vi "timestamp to string.vi"(7 "Return UTC":bool, 10 "Format":string(combo), 11 "time stamp":timestamp) -> (3 "date/time string":string)   [LabVIEW 2013]
panel:
  # "%^<%Y_%m_%d_T%H_%M_%S>T\n2011_01_11_T13_01_11\n%^<%Y_%m_%d_%H_%M_%S>T\n2011_01_11_13_01_11\n%^<%Y_%m_%d_T%H_%M_%S>T.txt\n2011_01_11_T13_01_11.txt\n\n%^<%b %d %Y %I:%M:%S %p>T\nJan 01 2012 01:01:11 PM\n%^<%b %d %Y %H:%M:%S>T\nJan 01 2012 13:01:11 \n%^<%a %d %b %Y %H:%M:%S>T\nSun 01 Jan 2012 13:01:11\n%^<%a %d %b %Y %I:%M:%S %p>T\nSun 01 Jan 2012 01:01:11 PM\n%^<%I:%M:%S %p %a %#m/%#d/%Y>T\n01:01:11 PM Sun 1/1/2012\n\n%^<%I:%M:%S %p>T\n01:01:11 PM\n%^<%H:%M:%S>T\n13:01:11\n%^<%a, %b %d %Y>T\nSun, Jan 01 2012\n%^<%d %b %Y>T\n01 Jan 2012"
  # "%^<%#I:%#M:%S %p %#m/%#d/%Y>T\n1:1:11 PM 1/11/2011 (USsmall TD)\n%^<%I:%M:%S %p %m/%d/%Y>T\n01:01:11 PM 01/11/2011 (USfull TD)\n\n%^<%#m/%#d/%Y %#I:%#M:%S %p>T\n1/11/2011 1:1:11 PM (USsmall DT)\n%^<%m/%d/%Y %I:%M:%S %p>T\n01/11/2011 01:01:11 PM(USfull DT)\n\n%^<%#H:%#M:%S %#d/%#m/%Y>T\n13:1:11 11/1/2011 (eurosmall TD)\n%^<%H:%M:%S %d/%m/%Y>T\n13:01:11 11/01/2011 (eurofull TD)\n\n%^<%#d/%#m/%Y %#H:%#M:%S>T\n13:1:11 11/1/2011 (eurosmall TD)\n%^<%d/%m/%Y %H:%M:%S>T\n13:01:11 11/01/2011 (eurofull TD)\n\n%^<%Y-%m-%d %H:%M:%S>T\n2011-11-01 13:01:11 (mysql datetime)"
  # "Time format codes have leading zeros as necessary to ensure a constant field width. An optional # modifier before the format code letter removes the leading zeros from the following format codes:\n\n%#d, %#H, %#I, %#j, %#m, %#M, %#s, %#S, %#U, %#w, %#W, %#X, %#y, %#Y\n\nDisplays a timestamp value or a numeric value as time in the format you specify using time format codes. For example, %c displays locale-specific date/time. Time-related format codes include the following: %X (locale-specific time), %H (hour, 24-hour clock), %I (hour, 12-hour clock), %M (minute), %S (second), %<digit>u (fractional seconds with <digit> precision), and %p (a.m./p.m. flag). Date-related format codes include the following: %x (locale-specific date), %y (year within century), %Y (year including century), %m (month number), %b (abbreviated month name), %d (day of month), and %a (abbreviated weekday name).\n%j day of year\n%W week of year\n%U full week of year\n%w day of week"
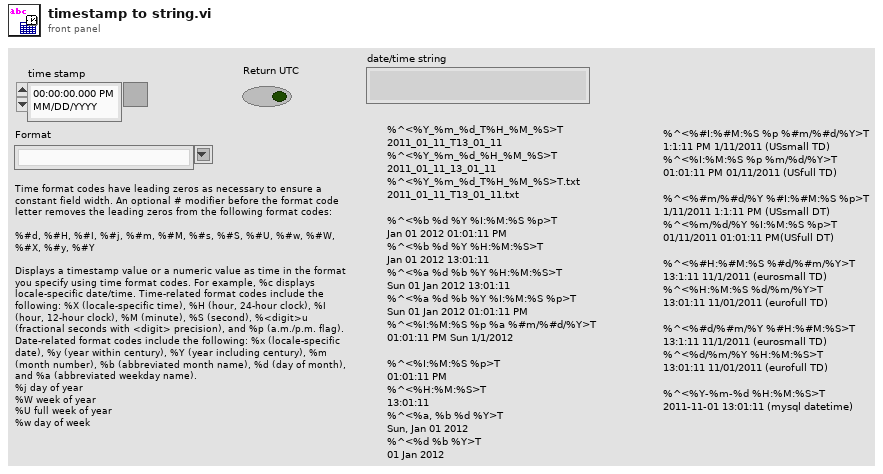
[diagram p1: front panel]
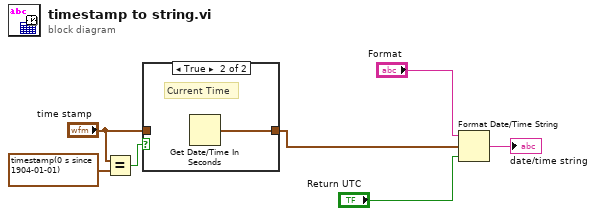
[diagram p0: block diagram]
diagram:
  n1 = Equal?(x="time stamp", y=timestamp(0 s since 1904-01-01) ("time stamp 2")) -> (x = y?=w6:bool)
  n2 = case shown="True" w6 {
    tunnel: [w8 w9] -> w5
    tunnel: "time stamp" -> [w8 _]
    frame False {
    }
    frame True {
      # "Current Time"
      n3 = Get Date/Time In Seconds() -> (seconds since 1Jan1904=w9:timestamp)
    }
  }
  n4 = Format Date/Time String(time format string (%c)="Format", seconds (now)=w5, UTC format="Return UTC") -> (date/time string=→"date/time string":string)
